vi "updatePanelFrame.vi"(8 "error in (no error)":errorcluster, 11 "UI in":refnum<class "UI.lvclass">) -> (0 "error out":errorcluster, 3 "UI out":refnum<class "UI.lvclass">)   [LabVIEW 2018, in "UI.lvclass"]
uses:
  UI.lvclass
  UI.lvclass/UI.ctl
  getPanel.vi
  getSubPanel.vi
  Panel/Panel.lvclass
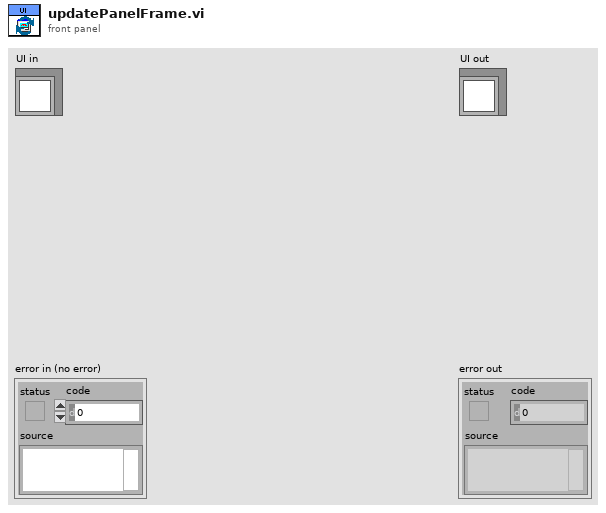
[diagram p1: front panel]
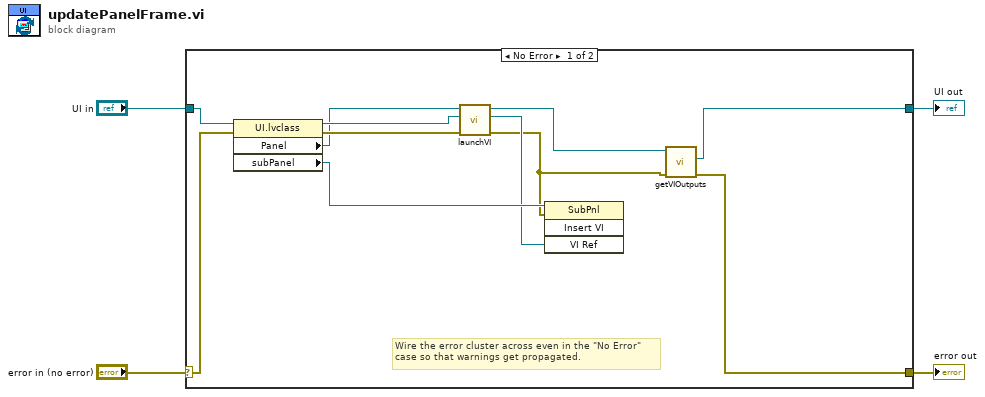
[diagram p0: block diagram]
diagram:
  n1 = case shown="No Error" "error in (no error)" {
    selector: "error in (no error)" -> [w14 w17]
    tunnel: [w11 w17] -> w3
    tunnel: [w10 w16] -> w1
    tunnel: "UI in" -> [w15 w16]
    frame No Error {
      # "Wire the error cluster across even in the \"No Error\"\ncase so that warnings get propagated."
      n2 = property class="UI.lvclass"(reference=w15, error in=w14) -> (reference out=w13:refnum<class "UI.lvclass">, error out=w12:errorcluster, "Panel"=w7:refnum<class "Panel.lvclass">, "subPanel"=w8:refnum<vi>)
      n3 = call "launchVI.vi"("error in (no error)"=w12, "UI.lvclass"=w13, "Panel in"=w7) -> ("error out"=w5:errorcluster, "VI ref Out"=w6:refnum<vi>, "Panel out"=w9:refnum<class "Panel.lvclass">)  [unwired: 6 in]
      n4 = invoke class="SubPnl" method="Insert VI"(reference=w8, error in=w5, "VI Ref"=w6) -> ()  [unwired: 1 in, 4 out]
      n5 = call "getVIOutputs.vi"("error in (no error)"=w5, "Panel in"=w9) -> ("error out"=w11:errorcluster, "UI.lvclass"=w10:refnum<class "UI.lvclass">)  [unwired: 7 in, 1 out]
    }
    frame Error {
    }
  }
  "error out" <- w3
  "UI out" <- w1
